vi "event driven state machine.vi"() -> ()   [LabVIEW 2018]
uses:
  State.ctl
panel:
  in  "Stop app":bool
  in  "Pause state machine":bool
  in  "Play state Machine":bool
  out "State":T1
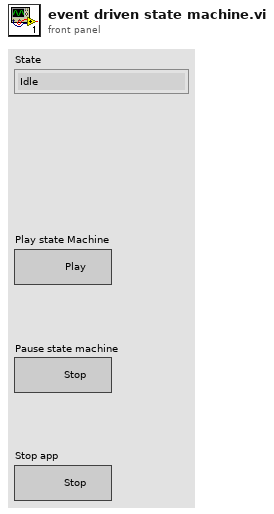
[diagram p1: front panel]
types:
  T1 = typedef "State.ctl" = enum16{"Idle", "Stop", "Play", "Init"}
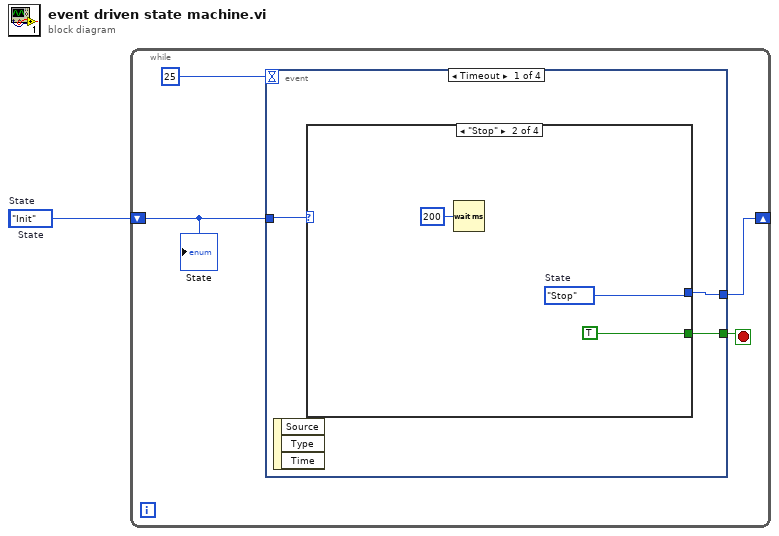
[diagram p0: block diagram]
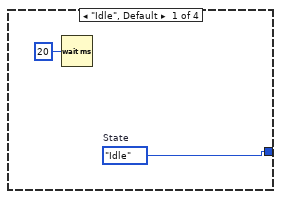
[diagram p2: hidden frame]
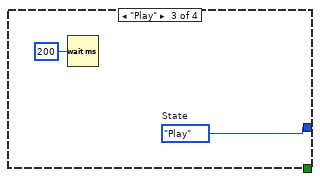
[diagram p3: hidden frame]
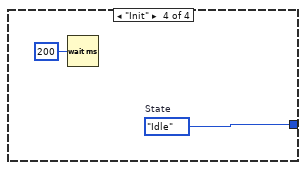
[diagram p4: hidden frame]
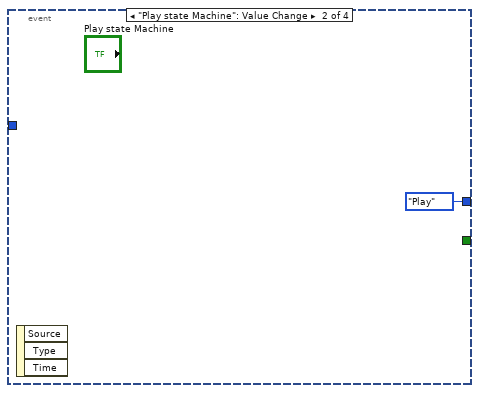
[diagram p5: hidden frame]
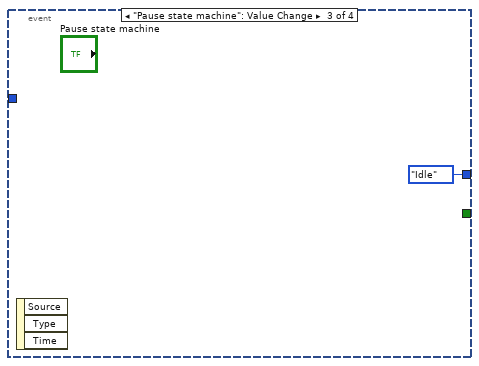
[diagram p6: hidden frame]
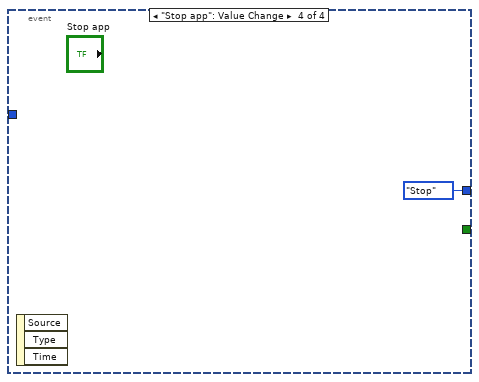
[diagram p7: hidden frame]
diagram:
  (unwired) State."Init"  # State
  w1 = State."Init"  # State
  n1 = while {
    shift-right: [w3] -> _
    shift-left: w1 -> [w4]
    stop <- w2 stop-if-true
    n2 = event shown="[0] Timeout" {
      selector: _ -> [_ _ _ _]
      dyn-events: _ -> [_ _ _ _]
      timeout: 25 -> [_ _ _ _]
      tunnel: w4 -> [w8 _ _ _]
      tunnel: [w7 State."Play" ("State") State."Idle" ("State") State."Stop" ("State")] -> w3
      tunnel: [w6 _ _ _] -> w2
      event Timeout {
        n3 = event-data() -> ()  [unwired: 1 in, 3 out]
        n4 = case shown="\"Stop\"" w8 {
          tunnel: [w9 w11 w14 w17] -> w7
          tunnel: [_ TRUE _ _] -> w6
          frame "Idle", Default {
            w9 = State."Idle"  # State
            n5 = Wait (ms)(milliseconds to wait=u32 20) -> ()  [unwired: 1 out]
          }
          frame "Stop" {
            w11 = State."Stop"  # State
            n6 = Wait (ms)(milliseconds to wait=u32 200) -> ()  [unwired: 1 out]
          }
          frame "Play" {
            w14 = State."Play"  # State
            n7 = Wait (ms)(milliseconds to wait=u32 200) -> ()  [unwired: 1 out]
          }
          frame "Init" {
            w17 = State."Idle"  # State
            n8 = Wait (ms)(milliseconds to wait=u32 200) -> ()  [unwired: 1 out]
          }
        }
      }
      event "Play state Machine": Value Change {
        n9 = event-data() -> ()  [unwired: 1 in, 3 out]
      }
      event "Pause state machine": Value Change {
        n10 = event-data() -> ()  [unwired: 1 in, 3 out]
      }
      event "Stop app": Value Change {
        n11 = event-data() -> ()  [unwired: 1 in, 3 out]
      }
    }
    "State" <- w4
  }
